vi "Decode Video (SubVI).vi"(11 "ImgData":u8[](array[numeric])) -> (2 "new picture":picture, 3 "Array":u32[][](array[numeric]))   [LabVIEW 2014]
uses:
  <vilib>/picture/picture.llb/Draw True-Color Pixmap.vi
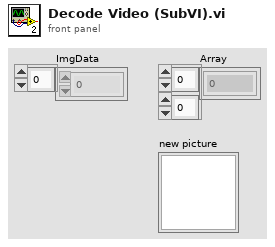
[diagram p1: front panel]
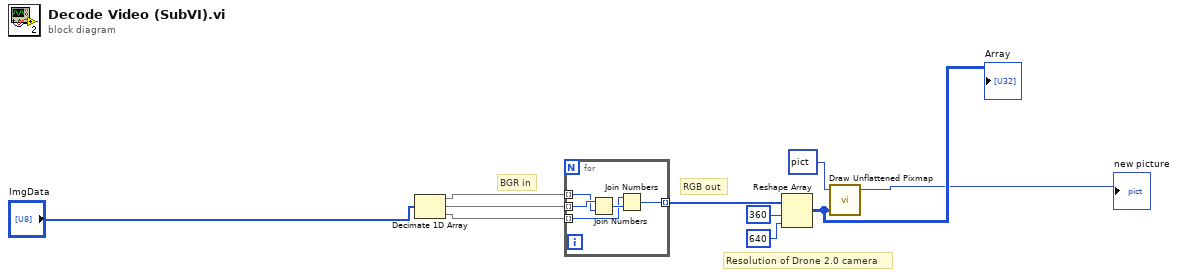
[diagram p0: block diagram]
diagram:
  # "Resolution of Drone 2.0 camera"
  # "RGB out"
  # "BGR in"
  n1 = Decimate 1D Array("ImgData") -> (w4:u8[], w5:u8[], w6:u8[])
  n2 = for {
    tunnel: [w14] -> w9 mode=indexing
    tunnel: w4 -> [w12] mode=indexing
    tunnel: w5 -> [w13] mode=indexing
    tunnel: w6 -> [w11] mode=indexing
    n3 = Join Numbers(hi=w13, lo=w12) -> ((hi.lo)=w15:u16)
    n4 = Join Numbers(hi=w11, lo=w15) -> ((hi.lo)=w14:u32)
  }
  n5 = Reshape Array(w9, 360 ("dimension size"), 640 ("dimension size")) -> (w10:u32[][])
  "Array" <- w10
  n6 = call-poly <vilib>:"Draw Unflattened Pixmap.vi"("picture"=picture data[5B], "data (RGB format)"=w10) -> ("new picture"=→"new picture":picture)  [unwired: 7 in]
